vi "JSON text to Variant (path).vi"(6 "LVClass Serializer":refnum<class "JSONtext LVClass Serializer.lvclass">, 7 "Item Path":string, 8 "error in (no error)":errorcluster, 9 "Variant (Data Type)":variant, 10 "Starting Offset":i32, 11 "JSON":string) -> (0 "error out":errorcluster, 1 "Variant out":variant, 3 "Found":bool)   [LabVIEW 2019, in "JSONtext.lvlib"]
uses:
  JSONtext.lvlib
  LVClass Serializer/JSONtext LVClass Serializer.lvclass
  String Subset.vi
  Parsing/Parse Full Path or Item Name.vi
  Next JSON Value.vi
  support/Error Cluster From Code.vi
  Offset/Find Item Locations by Path.vi
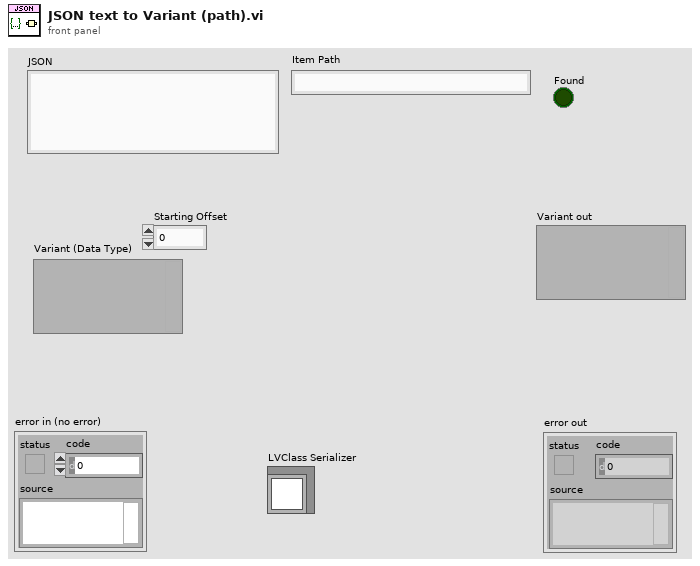
[diagram p1: front panel]
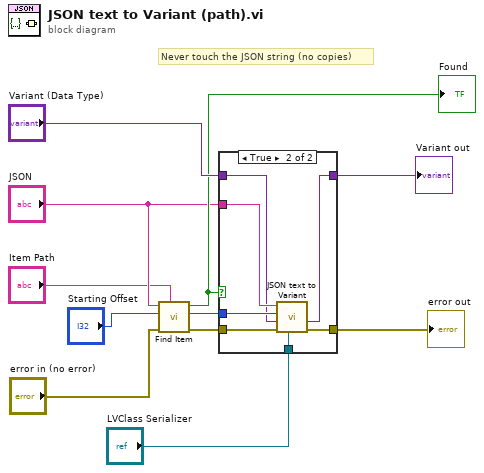
[diagram p0: block diagram]
diagram:
  # "Never touch the JSON string (no copies)"
  n1 = call "Find Item.vi"("$Path or Item Name"="Item Path", "error in (no error)"="error in (no error)", "Offset"="Starting Offset", "JSON"="JSON") -> ("error out"=w9:errorcluster, "Item offset"=w11:i32, "Found"=w5:bool)  [unwired: 4 in, 1 out]
  "Found" <- w5
  n2 = case shown="True" w5 {
    tunnel: "JSON" -> [_ w20]
    tunnel: w11 -> [_ w19]
    tunnel: w9 -> [w12 w18]
    tunnel: "Variant (Data Type)" -> [w13 w17]
    tunnel: [w12 w16] -> w7
    tunnel: [w13 w15] -> w6
    tunnel: "LVClass Serializer" -> [_ w14]
    frame False {
    }
    frame True {
      n3 = call "JSON text to Variant.vi"("LVClass Serializer"=w14, "error in (no error)"=w18, "Data Type"=w17, "Offset"=w19, "JSON"=w20) -> ("error out"=w16:errorcluster, "Variant out"=w15:variant)  [unwired: 5 in]
    }
  }
  "Variant out" <- w6
  "error out" <- w7
